vi "Self Test.vi"(8 "error in":errorcluster, 11 "3300 in":refnum<class "3300.lvclass">) -> (0 "error out":errorcluster, 3 "3300 out":refnum<class "3300.lvclass">)   [LabVIEW 2019, in "3300.lvlib" / "3300.lvclass"]
uses:
  Library/3300.lvclass
  Library/3300.lvclass/3300.ctl
  builds/Instruments/Electronic Load.lvlibp/Library/Electronic Load.lvclass
  <instrlib>/Agilent N330X Series/Agilent N330X Series.lvlib
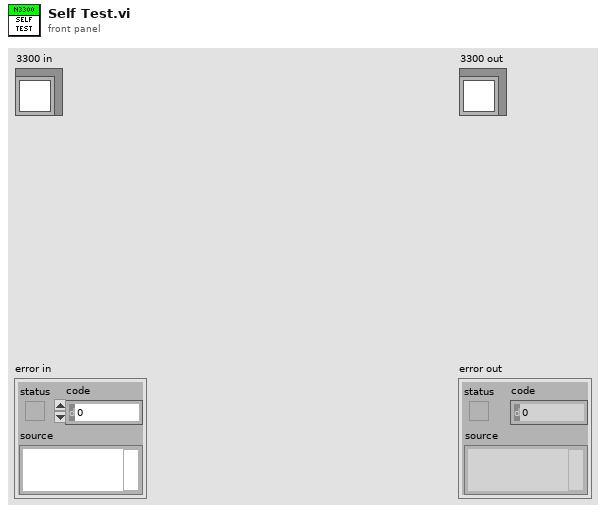
[diagram p1: front panel]
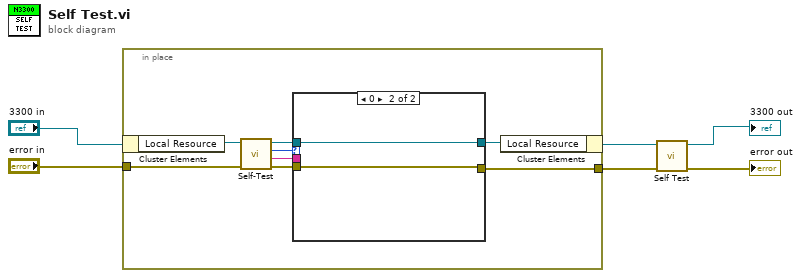
[diagram p0: block diagram]
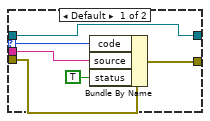
[diagram p2: hidden frame]
diagram:
  n1 = in-place {
    in-place-border: "error in" -> [w13]
    in-place-border: [w7] -> w3
    n2 = in-place-cluster #1("3300 in") -> ("Local Resource"=w14:refnum<visa-resource-name>)
    n3 = call <instrlib>:"Self-Test.vi"("error in (no error)"=w13, "VISA resource name"=w14) -> ("error out"=w11:errorcluster, "Self-Test Result Message"=w10:string, "Self-Test Result Code"=w9:i32, "VISA resource name out"=w12:refnum<visa-resource-name>)  [unwired: 6 in]
    n4 = case shown="0" w9 {
      selector: w9 -> [w19 _]
      tunnel: w12 -> [w16 w21]
      tunnel: w11 -> [w20 w22]
      tunnel: w10 -> [w18 _]
      tunnel: [w17 w22] -> w7
      tunnel: [w16 w21] -> w8
      frame Default {
        n5 = Bundle By Name(cluster=w20, "code"=w19, "source"=w18, "status"=TRUE) -> (w17:errorcluster)
      }
      frame 0 {
      }
    }
    n6 = in-place-cluster #1("Local Resource"=w8) -> (w4:refnum<class "3300.lvclass">)
  }
  n7 = call-parent "Self Test.vi"("error in"=w3, "Instruments in"=w4) -> ("error out"=→"error out":errorcluster, "Instruments out"=→"3300 out":refnum<class "3300.lvclass">)  [unwired: 8 in]
